vi "process_data_string.vi"(2 "error in (no error)":errorcluster, 3 "Data in":string) -> (0 "error out (no error)":errorcluster, 1 "Data out":string[](array[string]))   [LabVIEW 2011]
doc: "Process_data_string\n\nSplits the incoming string into an array of instrument strings. \n\n\nExamples:\n\ninstr1%instrdata1#instr2%instrdata2\n\nWill make an outgoing list of strings like:\ninstr1 instrdata1\ninstr2 instrdata2"
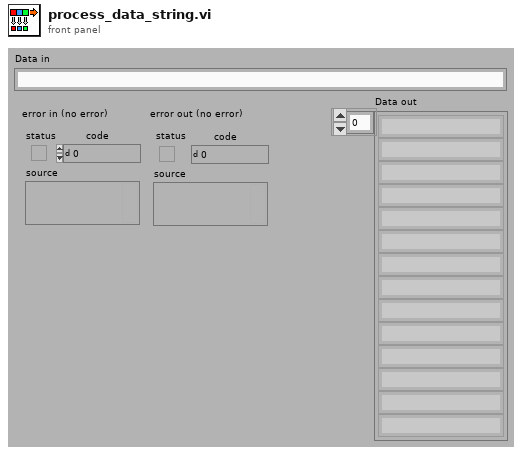
[diagram p1: front panel]
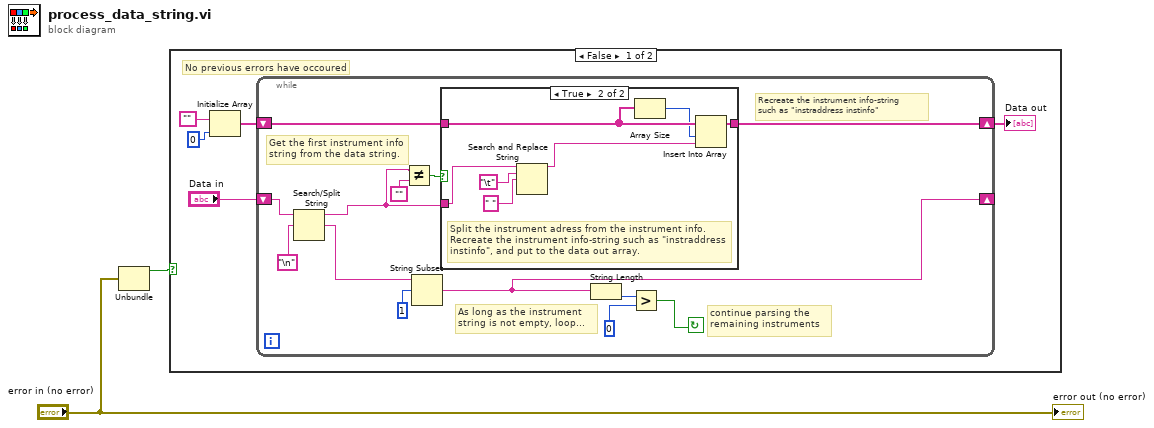
[diagram p0: block diagram]
diagram:
  n1 = Unbundle("error in (no error)") -> ("status"=w2:bool)  [unwired: 2 out]
  n2 = case shown="False" w2 {
    frame False {
      # "No previous errors have occoured"
      n3 = Initialize Array("", 0 ("dimension size")) -> (w5:string[])
      n4 = while {
        shift-left: w5 -> [w17]
        shift-right: [w16] -> w7
        shift-left: "Data in" -> [w15]
        shift-right: [w9] -> _
        stop <- w18 continue-if-true
        # "Recreate the instrument info-string\nsuch as \"instraddress instinfo\""
        # "As long as the instrument string is not empty, loop..."
        # "Get the first instrument info string from the data string."
        # "continue parsing the remaining instruments"
        n5 = Search/Split String(string=w15, search string/char (-)="\n") -> (substring before match=w11:string, match + rest of string=w13:string)  [unwired: 1 in, 1 out]
        n6 = Not Equal?(x=w11, y="") -> (x != y?=w12:bool)
        n7 = String Subset(string=w13, offset (0)=1) -> (substring=w9:string)  [unwired: 1 in]
        n8 = case shown="True" w12 {
          tunnel: w17 -> [w21 w27]
          tunnel: [w21 w28] -> w16
          tunnel: w11 -> [_ w25]
          frame False {
          }
          frame True {
            # "Split the instrument adress from the instrument info. Recreate the instrument info-string such as \"instraddress instinfo\", and put to the data out array."
            n9 = Search and Replace String(input string=w25, search string="\t" ("search string/char (-)"), replace string=" " ("string")) -> (result string=w22:string)  [unwired: 5 in, 3 out]
            n10 = Array Size(array=w27) -> (size(s)=w26:i32)
            n11 = Insert Into Array(array=w27, index=w26, new element=w22) -> (w28:string[])
          }
        }
        n12 = String Length(string=w9) -> (length=w20:i32)
        n13 = Greater?(x=w20, y=0) -> (0:w18:bool)
      }
      "Data out" <- w7
    }
    frame True {
      # "Previous errors have occoured!!!"
    }
  }
  "error out (no error)" <- "error in (no error)"
